vi "Resolve Group Conflicts.vi"(8 "error in (no error)":errorcluster, 9 "Current Group Number (0)":i32, 10 "Group Name in":string, 11 "TDMS Log File in":refnum<class "TDMS Log File.lvclass">) -> (0 "error out":errorcluster, 1 "Group Number":i32, 2 "Group Name out":string, 3 "TDMS Log File out":refnum<class "TDMS Log File.lvclass">)   [LabVIEW 2012, in "Waveform Data Logger Engine.lvlib" / "TDMS Log File.lvclass"]
uses:
  TDMS Log File.lvclass
  TDMS Log File.lvclass/TDMS Log File.ctl
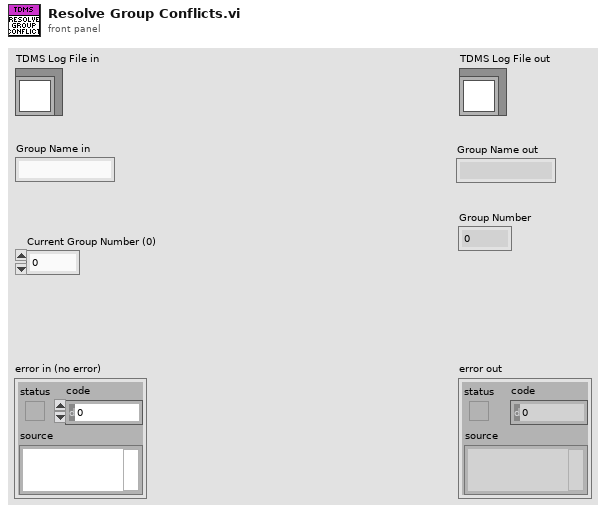
[diagram p1: front panel]
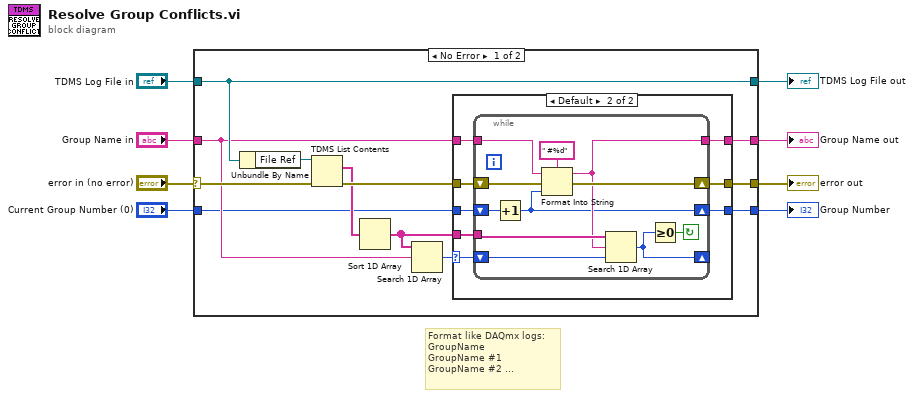
[diagram p0: block diagram]
diagram:
  # "Format like DAQmx logs:\nGroupName\nGroupName #1\nGroupName #2 ..."
  n1 = case shown="No Error" "error in (no error)" {
    selector: "error in (no error)" -> [w18 w45]
    tunnel: [w13 w45] -> w7
    tunnel: [w20 w44] -> w5
    tunnel: "TDMS Log File in" -> [w20 w44]
    tunnel: "Group Name in" -> [w16 w43]
    tunnel: [w15 w43] -> w3
    tunnel: "Current Group Number (0)" -> [w10 w42]
    tunnel: [w9 w42] -> w1
    frame No Error {
      n2 = Unbundle By Name(w20) -> ("File Ref"=w19:refnum<k34>)
      n3 = TDMS List Contents(4:w18, 7:w19) -> (0:w14:errorcluster, 2:w12:string[])  [unwired: 1 in, 2 out]
      n4 = Sort 1D Array(array=w12) -> (sorted array=w11:string[])
      n5 = Search 1D Array(1D array=w11, element=w16) -> (index of element=w17:i32)  [unwired: 1 in]
      n6 = case shown="Default" w17 {
        selector: w17 -> [_ w25]
        tunnel: w16 -> [w22 w28]
        tunnel: [w22 w27] -> w15
        tunnel: w14 -> [w21 w30]
        tunnel: w11 -> [_ w29]
        tunnel: [w21 w26] -> w13
        tunnel: w10 -> [_ w24]
        tunnel: [_ w23] -> w9
        frame -1 {
          # "Group does not\ncurrently exist in file.\nUse as-is."
        }
        frame Default {
          n7 = while {
            shift-right: [w36] -> w26
            shift-left: w30 -> [w41]
            tunnel: w29 -> [w38]
            tunnel: w28 -> [w39]
            tunnel: [w35] -> w27
            shift-right: [w33] -> _
            shift-left: w25 -> [w34]
            shift-right: [w31] -> w23
            shift-left: w24 -> [w32]
            stop <- w37 continue-if-true
            n8 = Increment(x=w32) -> (x+1=w31:i32)
            n9 = Format Into String(format string=" #%d", initial string=w39, error in=w41, w31) -> (resulting string=w35:string, error out=w36:errorcluster)
            n10 = Search 1D Array(1D array=w38, element=w35, start index (0)=w34) -> (index of element=w33:i32)
            n11 = Greater Or Equal To 0?(x=w33) -> (x >= 0?=w37:bool)
          }
        }
      }
    }
    frame Error {
    }
  }
  "error out" <- w7
  "TDMS Log File out" <- w5
  "Group Name out" <- w3
  "Group Number" <- w1
